vi "Bessel.vi"(1 "# terms":u16=10, 2 "order":u8=2, 3 "lambda":dbl[](array[numeric])=[1.0] format="%.2f") -> (0 "B (lambda":dbl[](array[numeric]) format="%.10f")   [LabVIEW 2018]
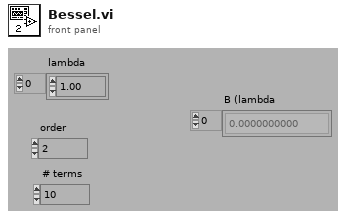
[diagram p1: front panel]
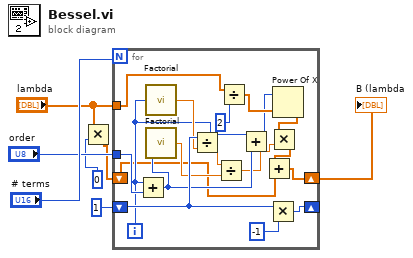
[diagram p0: block diagram]
diagram:
  n1 = Multiply(x="lambda", y=0) -> (x*y=w4:dbl[])
  n2 = for {
    N: "# terms" -> [_]
    tunnel: "lambda" -> [w17]
    shift-right: [w24] -> _
    shift-left: 1 -> [w22]
    tunnel: "order" -> [w23]
    shift-right: [w8] -> w1
    shift-left: w4 -> [w12]
    i -> [w15]
    n3 = Add(x=w15, y=w23) -> (x+y=w16:i32)
    n4 = call "Factorial.vi"("n"=w15) -> ("facgtorial"=w21:ext)
    n5 = call "Factorial.vi"("n"=w16) -> ("facgtorial"=w19:ext)
    n6 = Divide(x=w22, y=w21) -> (x/y=w20:ext)
    n7 = Divide(x=w20, y=w19) -> (x/y=w10:ext)
    n8 = Divide(x=w17, y=2) -> (x/y=w14:dbl[])
    n9 = Add(x=w15, y=w16) -> (x+y=w13:i32)
    n10 = Multiply(x=w22, y=-1) -> (x*y=w24:i32)
    n11 = Power Of X(1:w14, 2:w13) -> (0:w11:dbl[])
    n12 = Multiply(x=w11, y=w10) -> (x*y=w9:ext[])
    n13 = Add(x=w9, y=w12) -> (x+y=w8:ext[])
  }
  "B (lambda" <- w1
